vi "STAGE+mono+counter_edit8.vi"() -> ()   [LabVIEW 2017]
uses:
  Control 1.ctl
panel:
  out "XY Graph":cluster{dbl[], dbl[]}(graph)
  out "Waveform Graph":waveform(dbl)(graph) caption="Record 41  of  100"
  out "Waveform Graph 2":waveform(dbl)(graph) caption="Record 41  of  100"
  out "Slide":i32(slide) scale=0.0..100.0
  in  "?":enum32{"DELAY", "COUNTER", "MONO"}(tab)
  in  "Set this as t0":bool
  in  "Axis":i32=1
  in  "Motor ON":bool
  in  "Motor OFF":bool
  out "Current Position [mm]":dbl
  out "Final Position [mm]":dbl
  in  "Data Points":i32=100
  out "Current Point":i32
  in  "Step Size [um]":i32=10
  in  "Averaging Time [s]":dbl=0.1
  in  "Rep Rate [Hz]":dbl=500.0
  out "Shots":dbl
  in  "Target [mm]":dbl format="%.3f"
  in  "Move":bool
  out "Initial position [mm]":dbl
  in  "GPIB address":string="23"
  in  "Count Mode":u16(ring) items=["A,B for Preset T", "A-B for Preset T", "A+B for Preset T", "A for Preset B"]
  in  "Trigger mode":u16(ring) items=["10 MHz"=0, "Input 2"=2, "Input T"=3]
  in  "Channel A Input":u16(ring)=1 items=["10 MHz", "Input 1"]
  in  "Channel B Input":u16(ring)=2 items=["Input 1"=1, "Input 2"=2]
  in  "Number of Measurements\n to take at one point/ Number of Periods":u16=1 min=1 max=2000 step=1
  in  "Time between measurements\n at one point (s)/Dwell Time":dbl=0.002 min=0.002 max=60.0 step=0.001
  in  "gate A mode (CW:0)":i16(slide) scale=0.0..2.0 scale format="%.2f"
  out "Counts":i32
  in  "Integrating time, 10^-7 sec":dbl=10000000.0
  out "Mono port":T1(ring)
  out "Time delay":u32=450000 min=1
  out "Serial":u32=12345
  in  "Step size":dbl=10.0 min=0.0
  in  "Scan to":i32=4000
  in  "Scan from":i32=2600
  out "Current wavelength":dbl
  out "Grt#":u8=1 min=1 max=3 step=1
  in  "?":bool
  out "Groove/mm":u32=1200
  out "Blaze (nm)":u32=300
  out "Timeout 2":bool
  in  "?":bool
  out "Timeout":bool
  in  "Collect Data!":bool
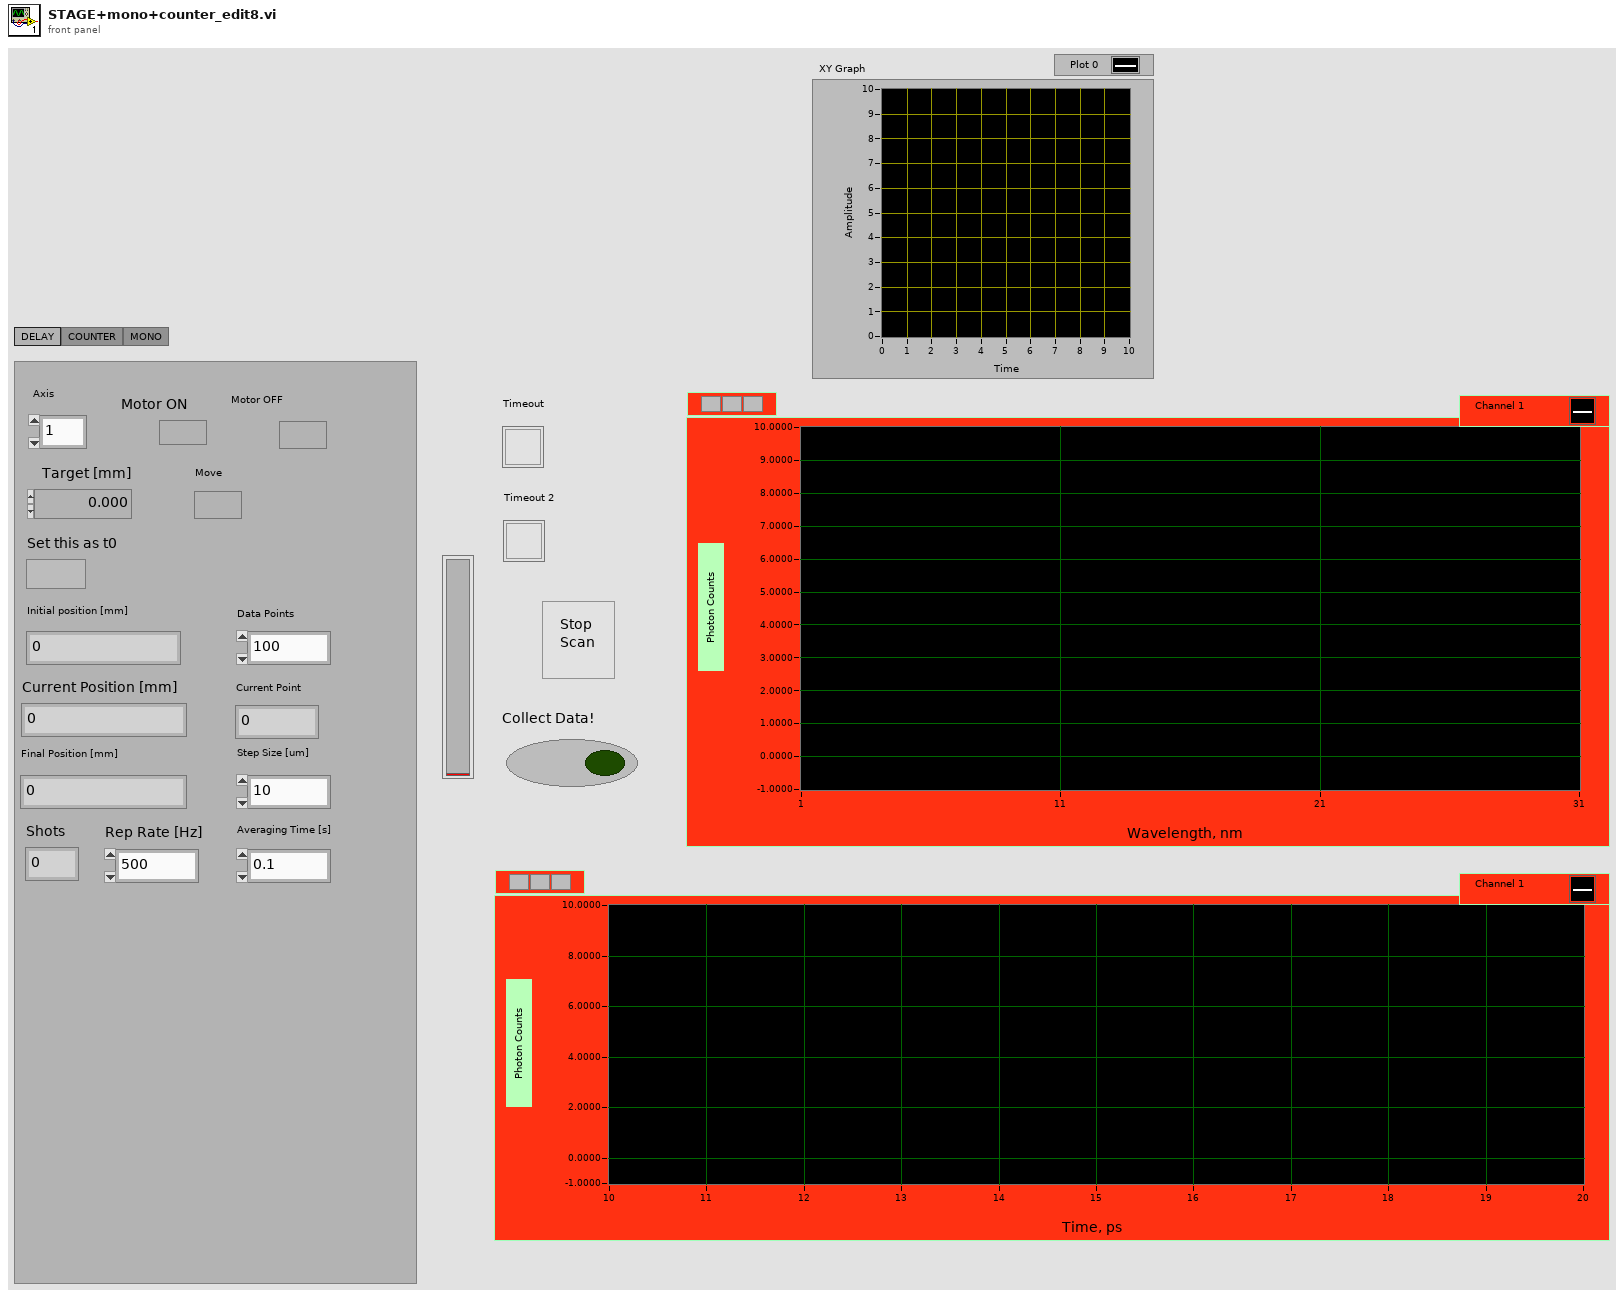
[diagram p1: front panel]
types:
  T1 = enum8{"COM 1", "COM 2", "COM 3", "COM 4", "COM 5", "COM 6", "COM 7", "COM 8", "COM 9"}
  T2 = cluster{"input XON/XOFF":bool, "input HW Handshake":bool, "input alt HW HShk":bool, "output XON/XOFF":bool, "output HW Handshake":bool, "output alt HW HShk":bool, "XOFF byte":u8, "XON byte":u8, "parity error byte":u16}
  T3 = enum16{"no parity", "odd parity", "even parity", "mark parity", "space parity"}
  T4 = typedef "Control 1.ctl" = dbl[]
  T5 = cluster{"Y[0]":dbl, "Y[1]":dbl, "Y[2]":dbl, "Y[3]":dbl, "Y[4]":dbl, "Y[5]":dbl, "Y[6]":dbl, "Y[7]":dbl, "Y[8]":dbl}
  T6 = typedef "NI_Matrix.lvlib/RealMatrix.ctl" = dbl[][]
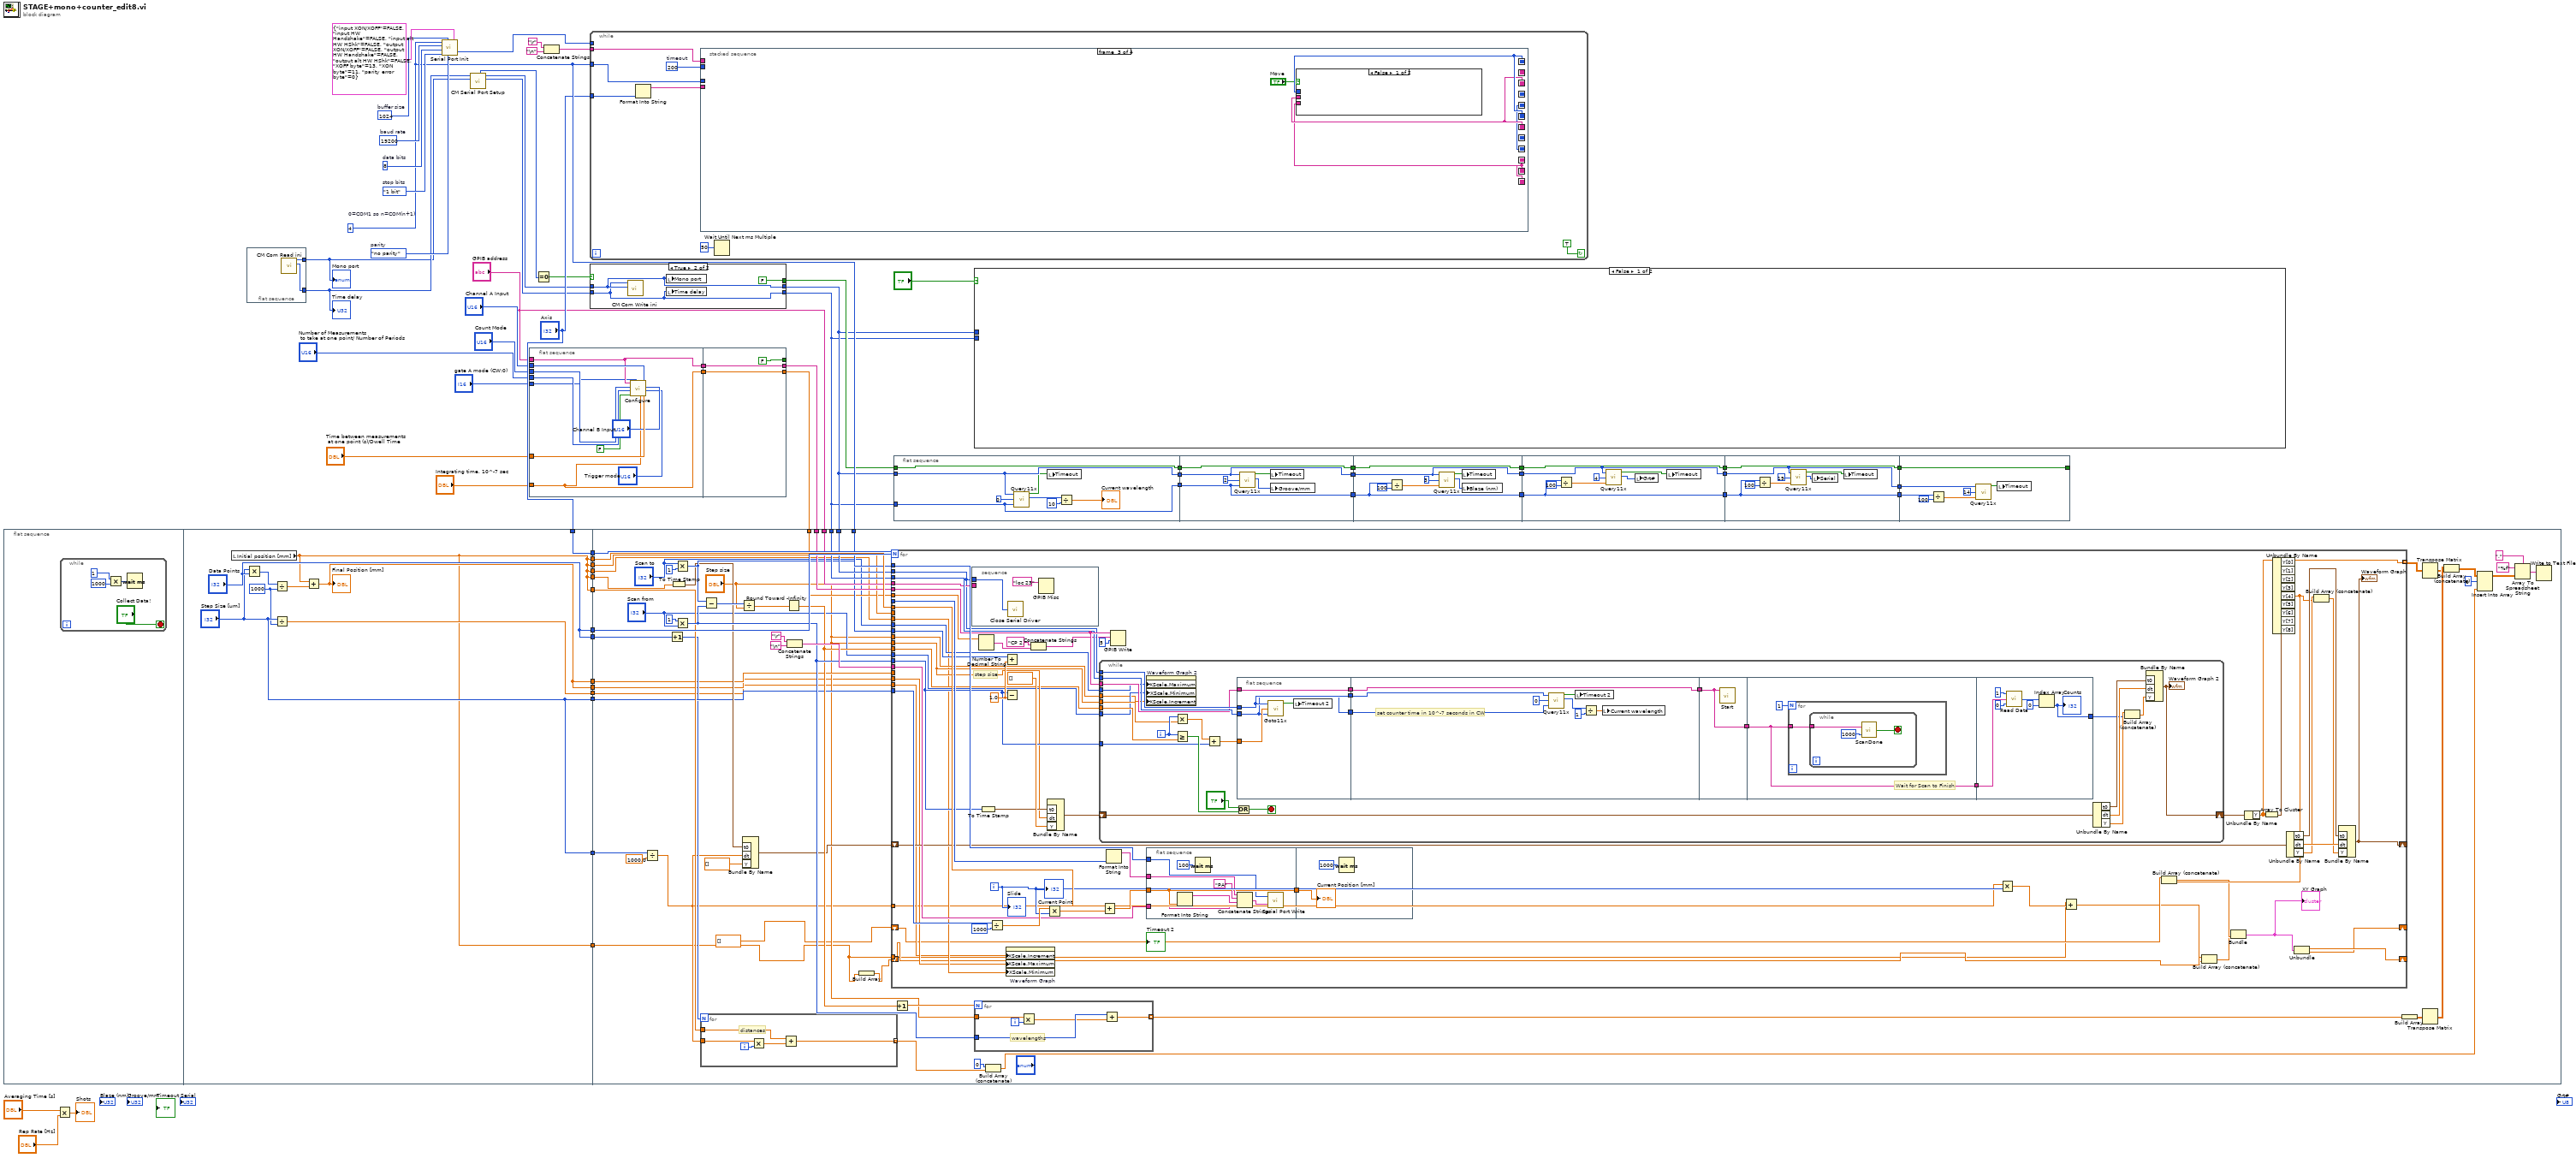
[diagram p0: block diagram]
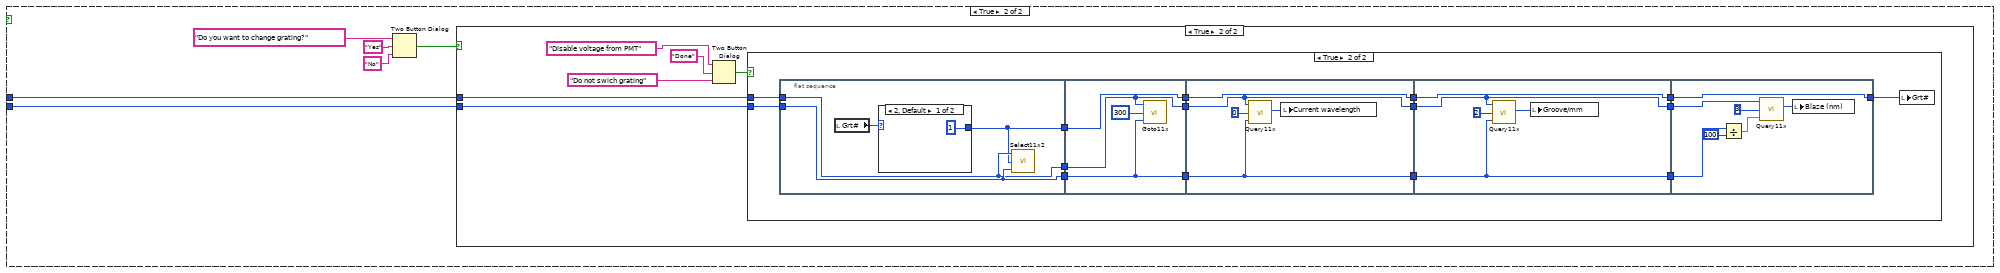
[diagram p2: hidden frame]
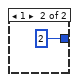
[diagram p5: hidden frame]
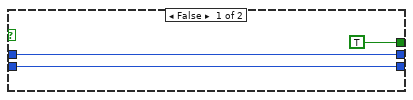
[diagram p6: hidden frame]
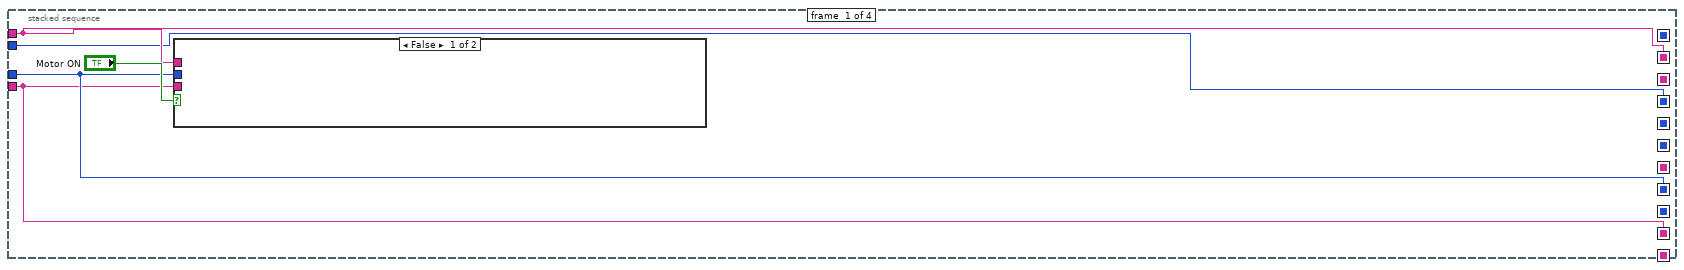
[diagram p7: hidden frame]
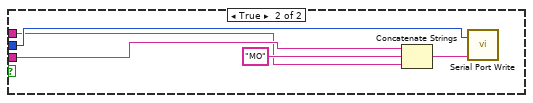
[diagram p8: hidden frame]
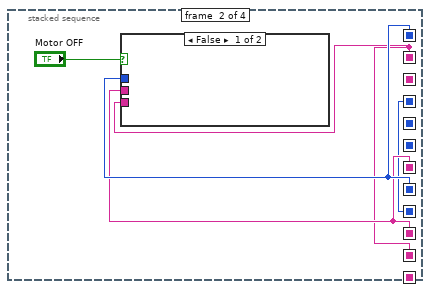
[diagram p9: hidden frame]
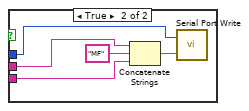
[diagram p10: hidden frame]
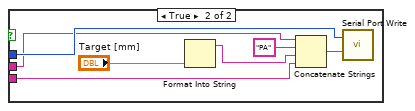
[diagram p11: hidden frame]
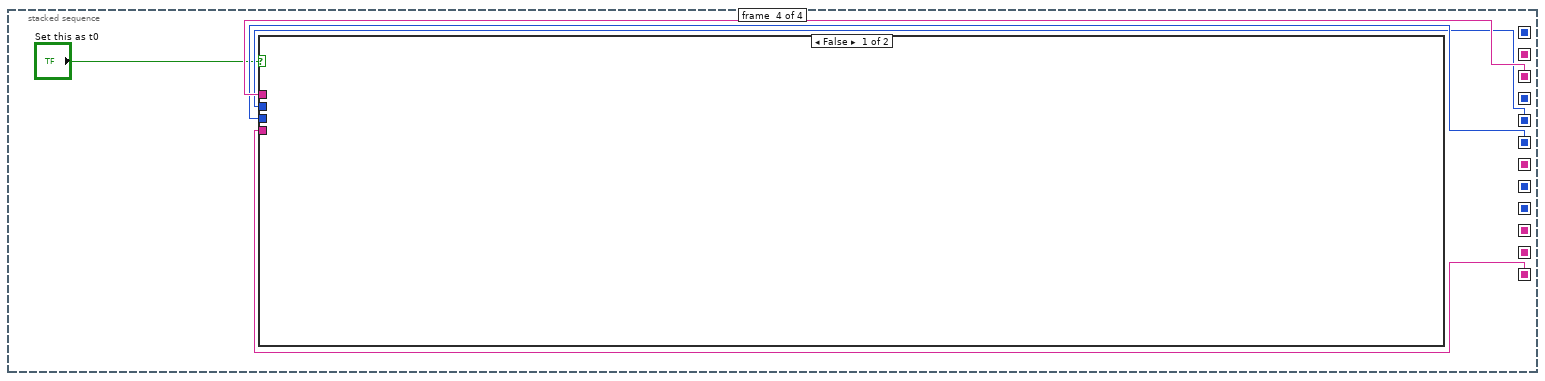
[diagram p12: hidden frame]
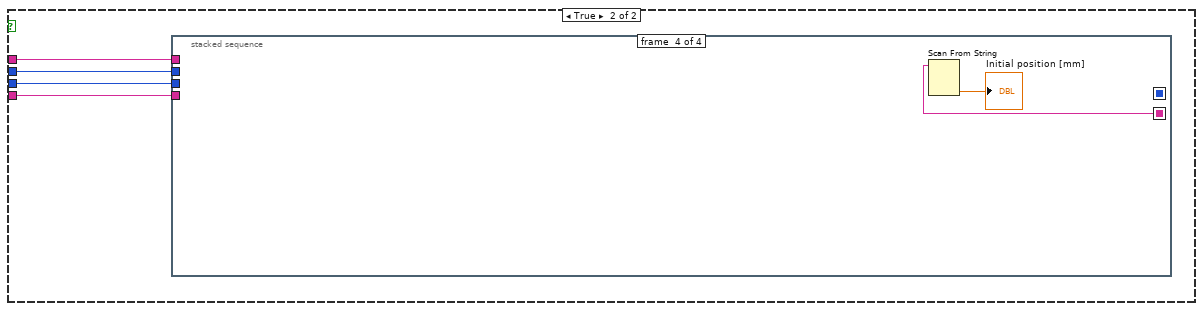
[diagram p13: hidden frame]
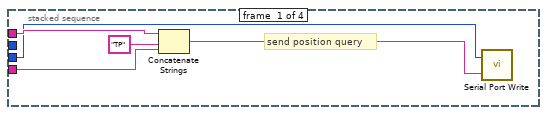
[diagram p14: hidden frame]
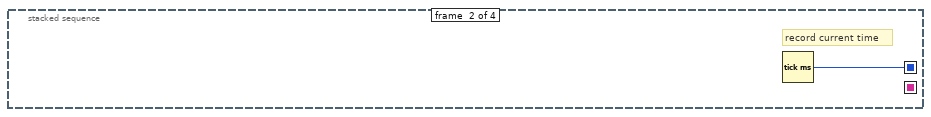
[diagram p15: hidden frame]
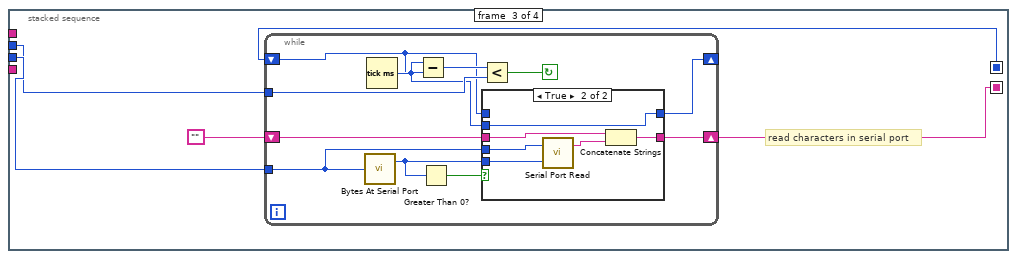
[diagram p16: hidden frame]
diagram:
  w56 = u32 19200  # baud rate
  w55 = u16 8  # data bits
  w54 = enum16{"1 bit", "1.5 bits", "2 bits"}."1 bit"  # stop bits
  w59 = T3."no parity"  # parity
  w53 = 4  # 0=COM1 so n=COM(n+1)
  w58 = u16 1024  # buffer size
  n1 = flat-sequence {
    tunnel: ["Data Points"] -> w65
    tunnel: "Axis" -> [w78]
    tunnel: [w70] -> w64
    tunnel: [w78] -> w63
    tunnel: [w70] -> w13
    tunnel: ["Step Size [um]"] -> w12
    tunnel: [w70] -> w11
    tunnel: ["Step Size [um]"] -> w10
    tunnel: ["Data Points"] -> w9
    tunnel: [w70] -> w8
    tunnel: [w74] -> w7
    tunnel: [w70] -> w4
    tunnel: [w74] -> w3
    tunnel: [w71] -> w2
    tunnel: [w70] -> w1
    tunnel: w65 -> [w134]
    tunnel: w64 -> [w133]
    tunnel: w63 -> [w132]
    tunnel: w53 -> [w128]
    tunnel: w17 -> [w127]
    tunnel: w16 -> [w126]
    tunnel: w15 -> [w125]
    tunnel: "GPIB address" -> [w124]
    tunnel: w13 -> [w107]
    tunnel: w12 -> [w106]
    tunnel: w11 -> [w101]
    tunnel: w10 -> [w100]
    tunnel: w9 -> [w98]
    tunnel: w8 -> [w91]
    tunnel: w7 -> [w90]
    tunnel: w6 -> [w89]
    tunnel: w4 -> [w85]
    tunnel: w3 -> [w84]
    tunnel: w2 -> [w83]
    tunnel: w1 -> [w79]
    frame #0 {
      n2 = while {
        stop <- "Collect Data!" stop-if-true
        n3 = Multiply(x=1, y=1000) -> (x*y=w69:i32)
        n4 = Wait (ms)(milliseconds to wait=w69) -> ()  [unwired: 1 out]
      }
    }
    frame #1 {
      w72 = 1000
      n5 = local read "Initial position [mm]"() -> (w70:dbl)
      n6 = Multiply(x="Step Size [um]", y="Data Points") -> (x*y=w77:i32)
      n7 = Divide(x=w77, y=w72) -> (x/y=w76:dbl)
      n8 = Divide(x="Step Size [um]", y=w72) -> (x/y=w71:dbl)
      n9 = Add(x=w70, y=w76) -> (x+y=w74:dbl)
      "Final Position [mm]" <- w74
    }
    frame #2 {
      n10 = Divide(x=w106, y=1000.0) -> (x/y=w82:dbl)
      n11 = Increment(x=w98) -> (x+1=w99:i32)
      n12 = To Time Stamp(1:w107) -> (0:w105:timestamp)
      n13 = Multiply(x="Scan to", y=1) -> (x*y=w118:i32)
      n14 = Multiply(x=1, y="Scan from") -> (x*y=w120:i32)
      n15 = for {
        N: w99 -> [_]
        tunnel: w82 -> [w139]
        tunnel: w101 -> [w137]
        tunnel: [w135] -> w97 mode=indexing
        i -> [w138]
        # "distances"
        n16 = Multiply(x=w139, y=w138) -> (x*y=w136:dbl)
        n17 = Add(x=w137, y=w136) -> (x+y=w135:dbl)
      }
      n18 = Subtract(x=w118, y=w120) -> (x-y=w117:i32)
      n19 = Divide(x=w117, y="Step size") -> (x/y=w116:dbl)
      n20 = Bundle By Name("t0"=w105, "dt"=w82, "Y"=T4 []) -> (w102:waveform(dbl))  [unwired: 1 in]
      n21 = Round Toward -Infinity(1:w116) -> (0:w115:dbl)
      n22 = Concatenate Strings("\r", "\n") -> (w129:string)
      n23 = Build Array(w79) -> (w80:dbl[])
      n24 = for {
        N: w134 -> [_]
        tunnel: w133 -> [w200]
        tunnel: w100 -> [w196]
        tunnel: w132 -> [w193]
        tunnel: w129 -> [w190]
        tunnel: w128 -> [w191]
        tunnel: w127 -> [w189]
        tunnel: w126 -> [w186]
        tunnel: w125 -> [w188]
        tunnel: w124 -> [w187]
        tunnel: [w172] -> w110 mode=indexing
        tunnel: w120 -> [w176]
        tunnel: w118 -> [w175]
        tunnel: "Step size" -> [w174]
        tunnel: w115 -> [w173]
        shift-right: [w164] -> _
        shift-left: w102 -> [w168]
        tunnel: w91 -> [_]
        tunnel: w90 -> [_]
        tunnel: w89 -> [w165]
        tunnel: "Scan to" -> [w163]
        tunnel: "Scan from" -> [w162]
        tunnel: "Step size" -> [w161]
        tunnel: w85 -> [w160]
        tunnel: w84 -> [w159]
        tunnel: w83 -> [w158]
        tunnel: w82 -> [w155]
        shift-right: [w154] -> _
        shift-left: w80 -> [w149]
        shift-right: [w151] -> _
        shift-left: T4 [] ("Y") -> [w150]
        tunnel: w79 -> [w148]
        i -> [w156]
        w185 = 1.0 ("x")
        # "step size"
        n25 = stacked-sequence {
          tunnel: w186 -> [w256]
          tunnel: w187 -> [_]
          frame #0 {
            n26 = call <vilib>:"Close Serial Driver.vi"("port number"=w256) -> ()  [unwired: 1 out]
            n27 = GPIB Misc(0:"loc 23" ("command string")) -> ()  [unwired: 1 in, 3 out]
          }
        }
        n28 = Number To Decimal String(number=w165) -> (decimal integer string=w180:string)  [unwired: 1 in]
        n29 = To Time Stamp(1:w176) -> (0:w183:timestamp)
        n30 = Divide(x=w196, y=1000) -> (x/y=w195:dbl)
        n31 = Add(x=w175, y=w185) -> ()  [unwired: 1 out]
        n32 = Subtract(x=w176, y=w185) -> ()  [unwired: 1 out]
        n33 = property on="Waveform Graph" class="WFGraph (strict)"("XScale.Increment"=w158, "XScale.Maximum"=w159, "XScale.Minimum"=w160) -> ()  [unwired: 2 in, 2 out]
        n34 = Concatenate Strings("CP 2,", w180) -> (w178:string)
        n35 = Multiply(x=w195, y=w156) -> (x*y=w199:dbl)
        n36 = Bundle By Name("t0"=w183, "dt"=w174, "Y"=dbl[] []) -> (w182:waveform(dbl))  [unwired: 1 in]
        n37 = while {
          tunnel: w186 -> [w227]
          tunnel: w188 -> [w226]
          shift-right: [w204] -> w177
          shift-left: w182 -> [w224]
          tunnel: w189 -> [w216]
          tunnel: w176 -> [w207]
          tunnel: w174 -> [w206]
          tunnel: w173 -> [w205]
          tunnel: w163 -> [w203]
          tunnel: w162 -> [w202]
          tunnel: w161 -> [w201]
          i -> [w221]
          stop <- w225 stop-if-true
          n38 = property on="Waveform Graph 2" class="WFGraph (strict)"("XScale.Maximum"=w203, "XScale.Minimum"=w202, "XScale.Increment"=w201) -> ()  [unwired: 2 in, 2 out]
          n39 = Multiply(x=w221, y=w206) -> (x*y=w228:dbl)
          n40 = Greater Or Equal?(x=w221, y=w205) -> (x >= y?=w217:bool)
          n41 = Add(x=w228, y=w207) -> (x+y=w208:dbl)
          n42 = Or(x="?", y=w217) -> (x .or. y?=w225:bool)
          n43 = flat-sequence {
            tunnel: w208 -> [w233]
            tunnel: w227 -> [w232]
            tunnel: [w232] -> w214
            tunnel: w226 -> [w231]
            tunnel: [w231] -> w213
            tunnel: w216 -> [w229]
            tunnel: [w229] -> w212
            tunnel: w214 -> [w240]
            tunnel: w213 -> [w239]
            tunnel: w212 -> [w237]
            tunnel: [w237] -> w211
            tunnel: w211 -> [w242]
            tunnel: [w242] -> w210
            tunnel: w210 -> [w243]
            tunnel: [w243] -> w209
            tunnel: w209 -> [w250]
            tunnel: [w249] -> w215
            frame #0 {
              n44 = call "Goto11x.vi"("time delay"=w231, "WAVELENGTH"=w233, "port number"=w232) -> ("timeout"=w230:bool)  [unwired: 2 out]
              n45 = local write "Timeout 2"(w230) -> ()
            }
            frame #1 {
              # "set counter time in 10^-7 seconds in CW"
              n46 = call "Query11x.vi"("port number"=w240, "QUERY"=0, "time delay"=w239) -> ("timeout"=w238:bool, "STATUS MESSAGE"=w236:u16)  [unwired: 2 out]
              n47 = local write "Timeout 2"(w238) -> ()
              n48 = Divide(x=w236, y=1) -> (x/y=w235:dbl)
              n49 = local write "Current wavelength"(w235) -> ()
            }
            frame #2 {
              n50 = call "Start.vi"("GPIB Address"=w242) -> ()  [unwired: 9 in]
            }
            frame #3 {
              # "Wait for Scan to Finish"
              n51 = for {
                N: 1 -> [_]
                tunnel: w243 -> [w245]
                n52 = while {
                  tunnel: w245 -> [w246]
                  stop <- w248 stop-if-true
                  n53 = call "ScanDone.vi"("Wait (ms)"=1000, "GPIB Address"=w246) -> ("Scan Finished?"=w248:bool)
                }
              }
            }
            frame #4 {
              n54 = call "Read Data.vi"("Channel Number"=0, "GPIB Address"=w250, "Number of Datapoints"=1) -> ("Data"=w251:i32[])
              n55 = Index Array(array=w251, index=0) -> (element=w249:i32)
              "Counts" <- w249
            }
          }
          n56 = Unbundle By Name(w224) -> ("t0"=w222:timestamp, "dt"=w223:dbl, "Y"=w220:dbl[])
          n57 = Build Array (concatenate)(w220, w215) -> (w219:dbl[])
          n58 = Bundle By Name("t0"=w222, "dt"=w223, "Y"=w219) -> (w204:waveform(dbl))  [unwired: 1 in]
          "Waveform Graph 2" <- w204
        }
        n59 = Add(x=w200, y=w199) -> (x+y=w198:dbl)
        n60 = Format Into String(w193) -> (resulting string=w192:string)  [unwired: 3 in, 1 out]
        n61 = GPIB Write(0:w189, 1:w178, 2:i16 5 ("mode (0)")) -> ()  [unwired: 2 in, 2 out]
        n62 = flat-sequence {
          tunnel: w198 -> [w259]
          tunnel: [w259] -> w194
          tunnel: w190 -> [w261]
          tunnel: w192 -> [w260]
          tunnel: w191 -> [w257]
          tunnel: w194 -> [w265]
          frame #0 {
            n63 = Format Into String(w259) -> (resulting string=w258:string)  [unwired: 3 in, 1 out]
            n64 = Wait (ms)(milliseconds to wait=u32 100) -> ()  [unwired: 1 out]
            n65 = Concatenate Strings(w260, "PA" ("Substring"), w258, w261) -> (w263:string)
            n66 = call <vilib>:"Serial Port Write.vi"("string to write"=w263, "port number"=w257) -> ()  [unwired: 1 out]
          }
          frame #1 {
            n67 = Wait (ms)(milliseconds to wait=u32 1000) -> ()  [unwired: 1 out]
            "Current Position [mm]" <- w265
          }
        }
        n68 = Multiply(x=w155, y=w156) -> (x*y=w157:dbl)
        n69 = Add(x=w148, y=w157) -> (x+y=w147:dbl)
        n70 = Build Array (concatenate)(w149, w147) -> (w146:dbl[])
        n71 = Unbundle By Name(w177) -> ("Y"=w172:dbl[])
        n72 = Array To Cluster(array=w172) -> (cluster=w171:T5)
        n73 = Unbundle By Name(w171) -> ("Y[4]"=w153:dbl)  [unwired: 8 out]
        n74 = Build Array (concatenate)(w150, w153) -> (w152:T4)
        n75 = Bundle(w146, "Y"=w152) -> (w145:cluster{dbl[], "Y":T4})  [unwired: 1 in]
        "XY Graph" <- w145
        n76 = Unbundle By Name(w168) -> ("t0"=w170:timestamp, "dt"=w169:dbl, "Y"=w167:dbl[])
        n77 = Unbundle(w145) -> (w154:dbl[], "Y"=w151:T4)
        n78 = Build Array (concatenate)(w167, w153) -> (w166:dbl[])
        n79 = Bundle By Name("t0"=w170, "dt"=w169, "Y"=w166) -> (w164:waveform(dbl))  [unwired: 1 in]
        "Waveform Graph" <- w164
        "Current Point" <- w156
        "Slide" <- w156
      }
      n80 = Increment(x=w115) -> (x+1=w114:dbl)
      n81 = for {
        N: w114 -> [_]
        tunnel: "Step size" -> [w144]
        tunnel: w120 -> [w142]
        tunnel: [w140] -> w112 mode=indexing
        i -> [w143]
        # "wavelengths"
        n82 = Multiply(x=w144, y=w143) -> (x*y=w141:dbl)
        n83 = Add(x=w142, y=w141) -> (x+y=w140:dbl)
      }
      n84 = Build Array (concatenate)(0, w97) -> (w94:dbl[])
      n85 = Build Array(w112) -> (w111:dbl[][])
      n86 = Transpose Matrix(1:w110) -> (0:w108:dbl[][])
      n87 = Transpose Matrix(1:w111) -> (0:w109:dbl[][])
      n88 = Build Array (concatenate)(w109, w108) -> (w93:T6)
      n89 = Insert Into Array(array=w93, index (row)=0, new element=w94) -> (w92:T6)  [unwired: 1 in]
      n90 = Array To Spreadsheet String(delimiter (Tab)=",", array=w92, 3:"%f" ("format string")) -> (spreadsheet string=w113:string)
      n91 = Write to Text File(text=w113) -> ()  [unwired: 3 in, 3 out]
    }
  }
  n92 = Multiply(x="Averaging Time [s]", y="Rep Rate [Hz]") -> (x*y=→"Shots":dbl)
  n93 = flat-sequence {
    tunnel: [w268] -> w31
    tunnel: [w267] -> w30
    frame #0 {
      n94 = call "CM Com Read ini.vi"() -> ("Mono port"=w267:T1, "time delay1"=w268:u32)  [unwired: 7 in]
    }
  }
  n95 = call <vilib>:"Serial Port Init.vi"("flow control etc."=T2 {"input XON/XOFF"=FALSE, "input HW Handshake"=FALSE, "input alt HW HShk"=FALSE, "output XON/XOFF"=FALSE, "output HW Handshake"=FALSE, "output alt HW HShk"=FALSE, "XOFF byte"=13, "XON byte"=11, "parity error byte"=0}, "parity"=w59, "buffer size"=w58, "stop bits"=w54, "data bits"=w55, "baud rate"=w56, "port number"=w53) -> ("error code"=w52:i32)
  n96 = call "CM Serial Port Setup.vi"("COM port"=w30, "time delay"=w31) -> ("time delay1"=w26:u32, "DK port Out"=w27:T1, "error code"=w29:i32)  [unwired: 7 in]
  n97 = flat-sequence {
    tunnel: "GPIB address" -> [w276]
    tunnel: [w276] -> w32
    tunnel: "Count Mode" -> [w277]
    tunnel: "Number of Measurements\n to take at one point/ Number of Periods" -> [w274]
    tunnel: "Time between measurements\n at one point (s)/Dwell Time" -> [w273]
    tunnel: "Channel A Input" -> [w278]
    tunnel: "gate A mode (CW:0)" -> [w270]
    tunnel: "Integrating time, 10^-7 sec" -> [w269]
    tunnel: [w269] -> w5
    tunnel: w32 -> [w280]
    tunnel: [w280] -> w17
    tunnel: [FALSE] -> _
    tunnel: [w279] -> w6
    tunnel: w5 -> [w279]
    frame #0 {
      n98 = call "Configure.vi"("Dwell Time (s)"=w273, "Channel T Input"="Trigger mode", "Channel B Input"="Channel B Input", "Channel A Input"=w278, "Integrating time, 10^-7 sec"=w269, "gate mode (CW:0)"=w270, "Scan End Mode"=FALSE, "Number of Periods"=w274, "Count Mode"=w277, "GPIB Address"=w276) -> ()
    }
    frame #1 {
    }
  }
  n99 = Equal To 0?(x=w29) -> (x = 0?=w28:bool)
  n100 = Concatenate Strings("\r", "\n") -> (w48:string)
  n101 = while {
    tunnel: w53 -> [w284]
    tunnel: w48 -> [w285]
    tunnel: w52 -> [_]
    tunnel: "Axis" -> [w282]
    stop <- TRUE continue-if-true
    w283 = u32 200  # timeout
    n102 = Format Into String(w282) -> (resulting string=w286:string)  [unwired: 3 in, 1 out]
    n103 = stacked-sequence {
      seq-local: [w291 _ _ _] -> [_ w302 _ _]
      seq-local: [w290 _ _ _] -> [_ w301 _ _]
      seq-local: [w292 _ _ _] -> [_ w303 _ _]
      seq-local: [w289 _ _ _] -> [_ w299 _ _]
      seq-local: [_ w302 _ _] -> [_ _ w312 _]
      seq-local: [_ w301 _ _] -> [_ _ w311 _]
      seq-local: [_ w303 _ _] -> [_ _ w313 _]
      seq-local: [_ w299 _ _] -> [_ _ w309 _]
      seq-local: [_ _ w312 _] -> [_ _ _ w325]
      seq-local: [_ _ w311 _] -> [_ _ _ w322]
      seq-local: [_ _ w313 _] -> [_ _ _ w324]
      seq-local: [_ _ w309 _] -> [_ _ _ w323]
      tunnel: w286 -> [w291 _ _ _]
      tunnel: w285 -> [w290 _ _ _]
      tunnel: w284 -> [w292 _ _ _]
      tunnel: w283 -> [w289 _ _ _]
      frame #0 {
        n104 = case shown="False" "Motor ON" {
          tunnel: w292 -> [_ w298]
          tunnel: w291 -> [_ w295]
          tunnel: w290 -> [_ w294]
          frame False {
          }
          frame True {
            n105 = Concatenate Strings(w295, "MO" ("Substring"), w294) -> (w296:string)
            n106 = call <vilib>:"Serial Port Write.vi"("string to write"=w296, "port number"=w298) -> ()  [unwired: 1 out]
          }
        }
      }
      frame #1 {
        n107 = case shown="False" "Motor OFF" {
          tunnel: w303 -> [_ w308]
          tunnel: w302 -> [_ w305]
          tunnel: w301 -> [_ w304]
          frame False {
          }
          frame True {
            n108 = Concatenate Strings(w305, "MF" ("Substring"), w304) -> (w306:string)
            n109 = call <vilib>:"Serial Port Write.vi"("string to write"=w306, "port number"=w308) -> ()  [unwired: 1 out]
          }
        }
      }
      frame #2 {
        n110 = case shown="False" "Move" {
          tunnel: w313 -> [_ w320]
          tunnel: w312 -> [_ w317]
          tunnel: w311 -> [_ w316]
          frame False {
          }
          frame True {
            n111 = Format Into String("Target [mm]") -> (resulting string=w314:string)  [unwired: 3 in, 1 out]
            n112 = Concatenate Strings(w317, "PA" ("Substring"), w314, w316) -> (w318:string)
            n113 = call <vilib>:"Serial Port Write.vi"("string to write"=w318, "port number"=w320) -> ()  [unwired: 1 out]
          }
        }
      }
      frame #3 {
        n114 = case shown="False" "Set this as t0" {
          tunnel: w325 -> [_ w329]
          tunnel: w324 -> [_ w328]
          tunnel: w323 -> [_ w327]
          tunnel: w322 -> [_ w326]
          frame False {
          }
          frame True {
            n115 = stacked-sequence {
              seq-local: [_ w335 _ _] -> [_ _ w337 _]
              seq-local: [_ _ w336 _] -> [_ _ _ w361]
              tunnel: w329 -> [w332 _ _ _]
              tunnel: w328 -> [w331 _ w340 _]
              tunnel: w327 -> [_ _ w338 _]
              tunnel: w326 -> [w330 _ _ _]
              frame #0 {
                # "send position query"
                n116 = Concatenate Strings(w332, "TP" ("Substring"), w330) -> (w333:string)
                n117 = call <vilib>:"Serial Port Write.vi"("string to write"=w333, "port number"=w331) -> ()  [unwired: 1 out]
              }
              frame #1 {
                # "record current time"
                n118 = Tick Count (ms)() -> (millisecond timer value=w335:u32)
              }
              frame #2 {
                # "read characters in serial port"
                n119 = while {
                  shift-left: w337 -> [w341]
                  shift-right: [w342] -> _
                  tunnel: w338 -> [w345]
                  shift-left: "" -> [w348]
                  shift-right: [w347] -> w336
                  tunnel: w340 -> [w349]
                  stop <- w344 continue-if-true
                  n120 = call <vilib>:"Bytes At Serial Port.vi"("port number"=w349) -> ("byte count"=w350:u32)  [unwired: 1 out]
                  n121 = Tick Count (ms)() -> (millisecond timer value=w343:u32)
                  n122 = Subtract(x=w343, y=w341) -> (x-y=w346:u32)
                  n123 = Greater Than 0?(x=w350) -> (x > 0?=w351:bool)
                  n124 = Less?(x=w346, y=w345) -> (x < y?=w344:bool)
                  n125 = case shown="True" w351 {
                    tunnel: w350 -> [_ w359]
                    tunnel: w349 -> [_ w358]
                    tunnel: w348 -> [w353 w356]
                    tunnel: [w353 w355] -> w347
                    tunnel: [w352 w354] -> w342
                    tunnel: w343 -> [_ w354]
                    tunnel: w341 -> [w352 _]
                    frame False {
                    }
                    frame True {
                      n126 = call <vilib>:"Serial Port Read.vi"("requested byte count"=w359, "port number"=w358) -> ("string read"=w357:string)  [unwired: 1 out]
                      n127 = Concatenate Strings(w356, w357) -> (w355:string)
                    }
                  }
                }
              }
              frame #3 {
                n128 = Scan From String(input string=w361) -> (output 1=→"Initial position [mm]":dbl)  [unwired: 4 in, 3 out]
              }
            }
          }
        }
      }
    }
    n129 = Wait Until Next ms Multiple(millisecond multiple=u32 50) -> ()  [unwired: 1 out]
  }
  n130 = case shown="True" w28 {
    tunnel: w27 -> [w364 w367]
    tunnel: w26 -> [w363 w366]
    tunnel: [w364 w367] -> w16
    tunnel: [w363 w366] -> w15
    tunnel: [TRUE FALSE] -> w25
    frame False {
    }
    frame True {
      n131 = call "CM Com Write ini.vi"("time delay1"=w367, "Mono port"=w366) -> ()  [unwired: 7 in]
      n132 = local write "Mono port"(w367) -> ()
      n133 = local write "Time delay"(w366) -> ()
    }
  }
  n134 = flat-sequence {
    tunnel: w15 -> [w373]
    tunnel: [w373] -> w47
    tunnel: w16 -> [w375]
    tunnel: [w375] -> w46
    tunnel: w25 -> [w371]
    tunnel: [w371] -> w45
    tunnel: w47 -> [w378]
    tunnel: [w378] -> w44
    tunnel: w46 -> [w380]
    tunnel: [w380] -> w43
    tunnel: w45 -> [w376]
    tunnel: [w376] -> w42
    tunnel: w44 -> [w388]
    tunnel: [w388] -> w41
    tunnel: w43 -> [w385]
    tunnel: [w385] -> w40
    tunnel: w42 -> [w382]
    tunnel: [w382] -> w39
    tunnel: w41 -> [w396]
    tunnel: [w396] -> w38
    tunnel: w40 -> [w393]
    tunnel: [w393] -> w37
    tunnel: w39 -> [w390]
    tunnel: [w390] -> w36
    tunnel: w38 -> [w404]
    tunnel: [w404] -> w35
    tunnel: w37 -> [w401]
    tunnel: [w401] -> w34
    tunnel: w36 -> [w398]
    tunnel: [w398] -> w33
    tunnel: w35 -> [w411]
    tunnel: w34 -> [w408]
    tunnel: [w406] -> _
    tunnel: w33 -> [w406]
    frame #0 {
      n135 = call "Query11x.vi"("port number"=w375, "QUERY"=u16 0, "time delay"=w373) -> ("timeout"=w372:bool, "STATUS MESSAGE"=w370:u16)  [unwired: 2 out]
      n136 = local write "Timeout"(w372) -> ()
      n137 = Divide(x=w370, y=10 ("Numeric")) -> (x/y=→"Current wavelength":dbl)
    }
    frame #1 {
      n138 = call "Query11x.vi"("port number"=w380, "QUERY"=u16 2, "time delay"=w378) -> ("timeout"=w377:bool, "STATUS MESSAGE"=w379:u16)  [unwired: 2 out]
      n139 = local write "Timeout"(w377) -> ()
      n140 = local write "Groove/mm"(w379) -> ()
    }
    frame #2 {
      n141 = Divide(x=w388, y=i16 100 ("device (1)")) -> (x/y=w386:dbl)
      n142 = call "Query11x.vi"("port number"=w385, "QUERY"=u16 3, "time delay"=w386) -> ("timeout"=w383:bool, "STATUS MESSAGE"=w384:u16)  [unwired: 2 out]
      n143 = local write "Timeout"(w383) -> ()
      n144 = local write "Blaze (nm)"(w384) -> ()
    }
    frame #3 {
      n145 = Divide(x=w396, y=i16 100 ("device (1)")) -> (x/y=w394:dbl)
      n146 = call "Query11x.vi"("port number"=w393, "QUERY"=u16 4, "time delay"=w394) -> ("timeout"=w391:bool, "STATUS MESSAGE"=w392:u16)  [unwired: 2 out]
      n147 = local write "Grt#"(w392) -> ()
      n148 = local write "Timeout"(w391) -> ()
    }
    frame #4 {
      n149 = Divide(x=w404, y=i16 100 ("device (1)")) -> (x/y=w402:dbl)
      n150 = call "Query11x.vi"("port number"=w401, "QUERY"=u16 19, "time delay"=w402) -> ("timeout"=w399:bool, "STATUS MESSAGE"=w400:u16)  [unwired: 2 out]
      n151 = local write "Serial"(w400) -> ()
      n152 = local write "Timeout"(w399) -> ()
    }
    frame #5 {
      n153 = Divide(x=w411, y=i16 100 ("device (1)")) -> (x/y=w409:dbl)
      n154 = call "Query11x.vi"("port number"=w408, "QUERY"=u16 14, "time delay"=w409) -> ("timeout"=w407:bool)  [unwired: 3 out]
      n155 = local write "Timeout"(w407) -> ()
    }
  }
  n156 = case shown="False" "?" {
    tunnel: w15 -> [_ w414]
    tunnel: w16 -> [_ w413]
    frame False {
    }
    frame True {
      n157 = Two Button Dialog(message="Do you want to change grating?", 1:"No" ("F button name (\"Cancel\")"), 2:"Yes" ("T button name (\"OK\")")) -> (T button?=w415:bool)
      n158 = case shown="True" w415 {
        tunnel: w414 -> [_ w420]
        tunnel: w413 -> [_ w419]
        frame False {
        }
        frame True {
          n159 = Two Button Dialog(message="Disable voltage from PMT", 1:"Do not swich grating" ("F button name (\"Cancel\")"), 2:"Done" ("T button name (\"OK\")")) -> (T button?=w421:bool)
          n160 = case shown="True" w421 {
            tunnel: w420 -> [_ w439]
            tunnel: w419 -> [_ w438]
            frame False {
            }
            frame True {
              n161 = flat-sequence {
                tunnel: w439 -> [w443]
                tunnel: [w443] -> w436
                tunnel: w438 -> [w442]
                tunnel: [w442] -> w435
                tunnel: [w440] -> w434
                tunnel: w436 -> [w447]
                tunnel: [w447] -> w433
                tunnel: w435 -> [w448]
                tunnel: [w448] -> w432
                tunnel: w434 -> [w446]
                tunnel: [w446] -> w431
                tunnel: w433 -> [w454]
                tunnel: [w454] -> w430
                tunnel: w432 -> [w453]
                tunnel: [w453] -> w429
                tunnel: w431 -> [w451]
                tunnel: [w451] -> w428
                tunnel: w430 -> [w457]
                tunnel: [w457] -> w427
                tunnel: w429 -> [w458]
                tunnel: [w458] -> w426
                tunnel: w428 -> [w455]
                tunnel: [w455] -> w425
                tunnel: w427 -> [w462]
                tunnel: w426 -> [w463]
                tunnel: [w460] -> w437
                tunnel: w425 -> [w460]
                frame #0 {
                  n162 = local read "Grt#"() -> (w441:u8)
                  n163 = case shown="2, Default" w441 {
                    tunnel: [1 2] -> w440
                    frame 2, Default {
                    }
                    frame 1 {
                    }
                  }
                  n164 = call "Select11x2.vi"("time delay"=w443, "NEW GRT?"=w440, "port number"=w442) -> ()  [unwired: 3 out]
                }
                frame #1 {
                  n165 = call "Goto11x.vi"("time delay"=w447, "WAVELENGTH"=u16 300, "port number"=w448) -> ()  [unwired: 3 out]
                }
                frame #2 {
                  n166 = call "Query11x.vi"("port number"=w453, "QUERY"=u16 0, "time delay"=w454) -> ("STATUS MESSAGE"=w450:u16)  [unwired: 3 out]
                  n167 = local write "Current wavelength"(w450) -> ()
                }
                frame #3 {
                  n168 = call "Query11x.vi"("port number"=w458, "QUERY"=u16 2, "time delay"=w457) -> ("STATUS MESSAGE"=w456:u16)  [unwired: 3 out]
                  n169 = local write "Groove/mm"(w456) -> ()
                }
                frame #4 {
                  n170 = Divide(x=w462, y=i16 100 ("device (1)")) -> (x/y=w464:dbl)
                  n171 = call "Query11x.vi"("port number"=w463, "QUERY"=u16 3, "time delay"=w464) -> ("STATUS MESSAGE"=w461:u16)  [unwired: 3 out]
                  n172 = local write "Blaze (nm)"(w461) -> ()
                }
              }
              n173 = local write "Grt#"(w437) -> ()
            }
          }
        }
      }
    }
  }
  "Mono port" <- w30
  "Time delay" <- w31
